vi "rqcBob Configure PD Detect FIFO (1PD PD1).vi"(8 "error in":errorcluster, 9 "PD.detect fifo depth":u32=1000000, 10 "PD.detect fifo write enable":bool, 11 "FPGA reference in":refnum<k20>) -> (0 "error out":errorcluster, 3 "FPGA reference out":refnum<k20>)   [LabVIEW 2018]
uses:
  <vilib>/Utility/error.llb/Error Cluster From Error Code.vi
  <vilib>/rvi/errors/niLvFpgaAdjustHostInterfaceError.vi
  <vilib>/rvi/interface/common/niFpgaWaitOnOcc.vi
  <vilib>/rvi/interface/nirviReadWriteControl/nirviReadWriteControl.xnode
  <vilib>/rvi/interface/nirviMethod/nirviMethod.xnode
  <vilib>/rvi/errors/niLvFpgaMergeErrorWithErrorCode.vi
  <vilib>/FPGAPlugInAG/Dynamic/niLvFpga_StartFifo_Dynamic.vi
  <vilib>/FPGAPlugInAG/Dynamic/niLvFpga_ConfigureFifo_Dynamic.vi
  NiFpgaLv.dll
  <vilib>/rvi/interface/Simulation/niFpgaSimulationCallBeginRW.vi
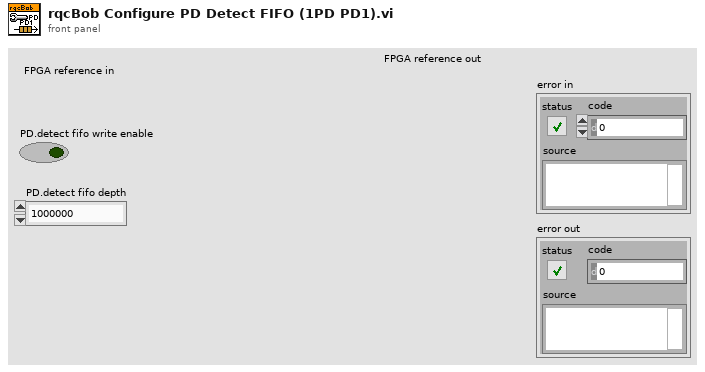
[diagram p1: front panel]
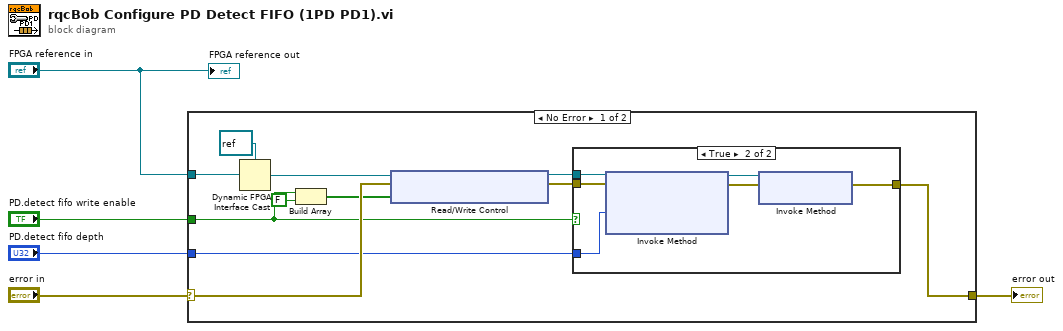
[diagram p0: block diagram]
diagram:
  n1 = case shown="No Error" "error in" {
    selector: "error in" -> [w16 w24]
    tunnel: [w10 w24] -> w3
    tunnel: "FPGA reference in" -> [w14 _]
    tunnel: "PD.detect fifo write enable" -> [w7 _]
    tunnel: "PD.detect fifo depth" -> [w9 _]
    frame No Error {
      n2 = Dynamic FPGA Interface Cast(Session In=refnum<k20> refnum ("FPGA Interface"), Type=w14) -> (Session Out=w13:refnum<k20>)
      n3 = Build Array(w7, FALSE ("element")) -> (w8:bool[])
      n4 = xnode "Read/Write Control"("FPGA VI Reference In"=w13, "error in"=w16, "PD.detect fifo write enable"=w8) -> ("FPGA VI Reference Out"=w12:refnum<k20>, "error out"=w11:errorcluster)
      n5 = case shown="True" w7 {
        tunnel: w12 -> [_ w23]
        tunnel: w11 -> [w17 w22]
        tunnel: [w17 w18] -> w10
        tunnel: w9 -> [_ w21]
        frame False {
        }
        frame True {
          n6 = xnode "Invoke Method"("FPGA VI Reference In"=w23, "error in"=w22, "Requested Depth"=w21) -> ("FPGA VI Reference Out"=w20:refnum<k20>, "error out"=w19:errorcluster)  [unwired: 1 out]
          n7 = xnode "Invoke Method"("FPGA VI Reference In"=w20, "error in"=w19) -> ("error out"=w18:errorcluster)  [unwired: 1 out]
        }
      }
    }
    frame Error {
    }
  }
  "error out" <- w3
  "FPGA reference out" <- "FPGA reference in"
